vi "GetPowerN1911a.vi"(6 "error in (no error)":errorcluster) -> (0 "Error out":errorcluster, 3 "Power returned (dBm)":dbl format="%#.10f")   [LabVIEW 2009]
doc: "Reads the power from the N1911A power meter."
panel:
  # "Get AVER power from N1911A insure that calc1:feed1 is set to AVER)"
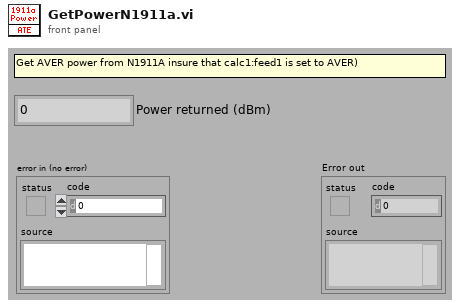
[diagram p1: front panel]
types:
  T1 = enum16{"N1911A", "Siggen", "34980a", "E4418B", "Rvp8"}
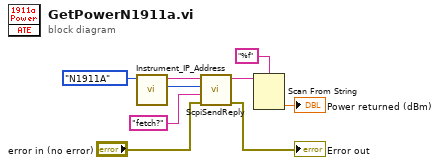
[diagram p0: block diagram]
diagram:
  n1 = call "Instrument_IP_Address.vi"("Instrument"=T1."N1911A") -> ("Port"=w1:u16, "IP Address"=w2:string)  [unwired: 9 in]
  n2 = call "ScpiSendReply.vi"("error in (no error)"="error in (no error)", "Command"="fetch?" ("format string"), "TCP port"=w1, "IP Address"=w2) -> ("Error out"=→"Error out":errorcluster, "Reply"=w7:string)  [unwired: 5 in]
  n3 = Scan From String(format string="%f", input string=w7) -> (output 1=→"Power returned (dBm)":dbl)  [unwired: 3 in, 3 out]
